vi "Zero_Degauss Current Probe.vi"() -> ()   [LabVIEW 2025, in "RIGOL MHO900 Series.lvlib"]
uses:
  RIGOL MHO900 Series.lvlib
panel:
  in  "Channel Name (0: Channel 1)":u16(ring) items=["Channel 1", "Channel 2", "Channel 3", "Channel 4"]
  out "VISA resource name out":refnum<visa-resource-name>
  out "error out":errorcluster
  in  "error in (no error)":errorcluster
  in  "VISA resource name":refnum<visa-resource-name>
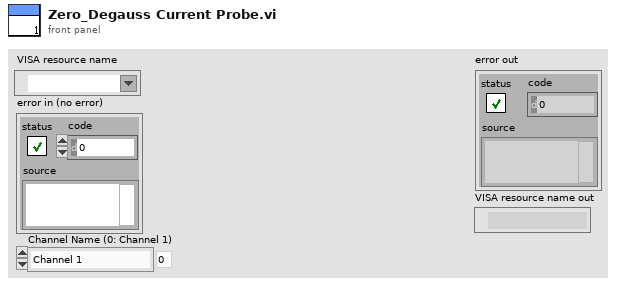
[diagram p1: front panel]
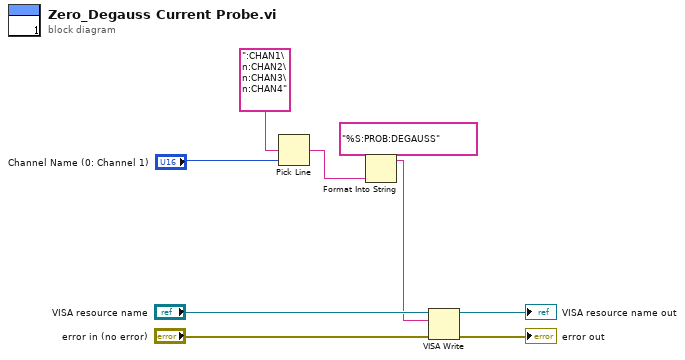
[diagram p0: block diagram]
diagram:
  n1 = Pick Line(multi-line string=":CHAN1\n:CHAN2\n:CHAN3\n:CHAN4", line index="Channel Name (0: Channel 1)") -> (output string=w2:string)  [unwired: 1 out]
  n2 = Format Into String(format string="%S:PROB:DEGAUSS", w2) -> (resulting string=w6:string)  [unwired: 2 in, 1 out]
  n3 = VISA Write(VISA resource name="VISA resource name", write buffer=w6, error in (no error)="error in (no error)") -> (VISA resource name out=→"VISA resource name out":refnum<visa-resource-name>, error out=→"error out":errorcluster)  [unwired: 1 out]
